vi "Trigger.vi"(8 "error in (no error)":errorcluster, 11 "Ni-Scope Digitizer in":refnum<class "Ni-Scope Digitizer.lvclass">) -> (0 "error out":errorcluster, 3 "Ni-Scope Digitizer out":refnum<class "Ni-Scope Digitizer.lvclass">)   [LabVIEW 2016, in "Ni-Scope Digitizer.lvclass"]
uses:
  Ni-Scope Digitizer.lvclass
  Ni-Scope Digitizer.lvclass/Ni-Scope Digitizer.ctl
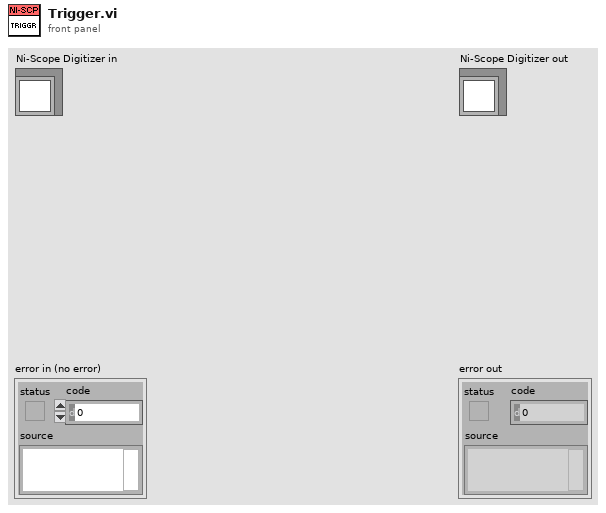
[diagram p1: front panel]
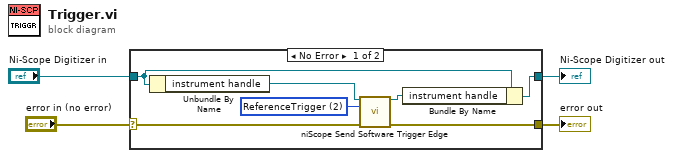
[diagram p0: block diagram]
diagram:
  n1 = case shown="No Error" "error in (no error)" {
    selector: "error in (no error)" -> [w9 w13]
    tunnel: "Ni-Scope Digitizer in" -> [w7 w12]
    tunnel: [w8 w13] -> w2
    tunnel: [w5 w12] -> w1
    frame No Error {
      w10 = u16 2 items=["StartTrigger", "ArmReferenceTrigger", "ReferenceTrigger", "AdvanceTrigger"] ("which trigger")
      n2 = Unbundle By Name(w7) -> ("instrument handle"=w11:refnum<k15>)
      n3 = call <instrlib>:"niScope Send Software Trigger Edge.vi"("instrument handle"=w11, "which trigger"=w10, "error in"=w9) -> ("instrument handle out"=w6:refnum<k15>, "error out"=w8:errorcluster)  [unwired: 11 in]
      n4 = Bundle By Name(cluster=w7, "instrument handle"=w6) -> (w5:refnum<class "Ni-Scope Digitizer.lvclass">)
    }
    frame Error {
    }
  }
  "error out" <- w2
  "Ni-Scope Digitizer out" <- w1
